vi "motionmenu.vi"(8 "Elements":string[](array[string]), 11 "NXT/EV3 2":T1) -> (0 "Goto":dbl, 1 "Continue?":bool, 3 "NXT/EV3":T1)   [LabVIEW 2013]
uses:
  <vilib>/NXT/Subs/LVHSConnector.ctl
  <vilib>/NXT/LegoClasses/BrickReference/BrickReference.lvclass
  <vilib>/NXT/Dual Mode Library/Waits/Wait_Num.vi
  <vilib>/NXT/Dual Mode Library/Display/clearDisplay.vi
  <vilib>/NXT/Dual Mode Library/Display/drawPicture.vi
  <vilib>/NXT/Dual Mode Library/Advanced/NXTFlag_Get.vi
  <vilib>/NXT/Dual Mode Library/Advanced/NXTFlag_Clear.vi
  <vilib>/NXT/Dual Mode Library/Advanced/NXTFlag_Get_Integer.vi
  <vilib>/NXT/Dual Mode Library/Sensors/EV3_Ultrasonic_CM.vi
  <vilib>/NXT/Dual Mode Library/Display/drawText_Center.vi
  <vilib>/NXT/Dual Mode Library/Advanced/NXTFlag_Assign.vi
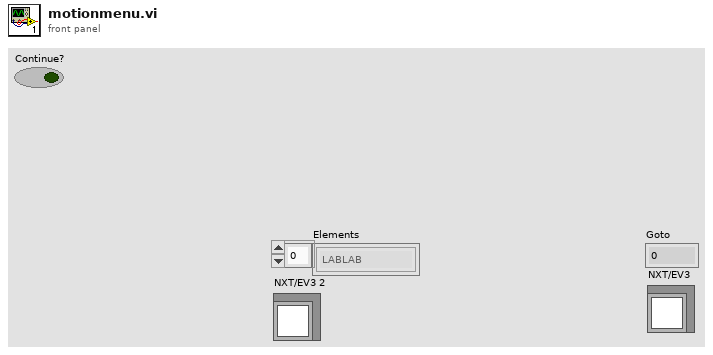
[diagram p1: front panel]
types:
  T1 = typedef "LVHSConnector.ctl" = refnum<class "BrickReference.lvclass">
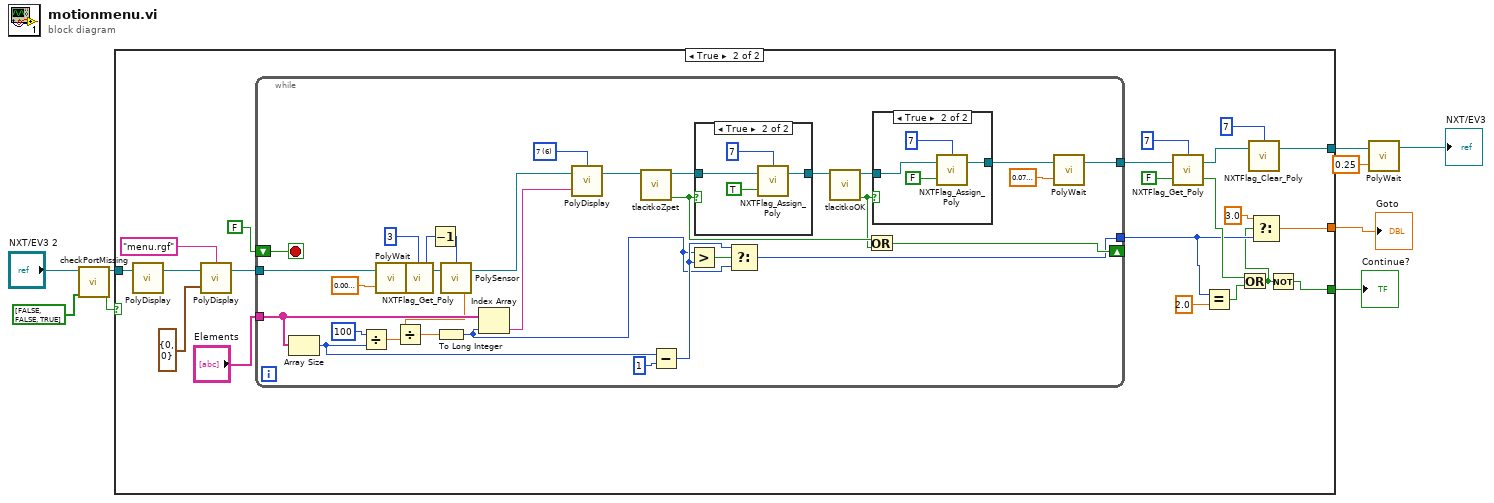
[diagram p0: block diagram]
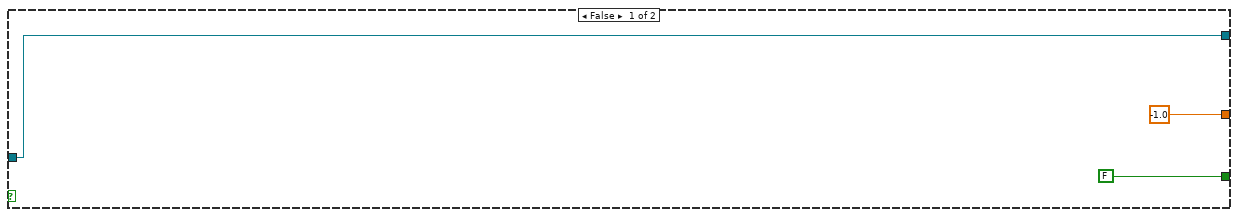
[diagram p2: hidden frame]
diagram:
  n1 = call "checkPortMissing.vi"("Required"=bool[] [FALSE, FALSE, TRUE], "NXT/EV3"="NXT/EV3 2") -> ("Success"=w4:bool, "NXT/EV3"=w6:T1)  [unwired: 8 in]
  n2 = case shown="True" w4 {
    tunnel: [-1.0 ("t") w18] -> w9
    tunnel: [w12 w21] -> w7
    tunnel: w6 -> [w12 w20]
    tunnel: [FALSE ("Boolean") w16] -> w3
    frame False {
    }
    frame True {
      n3 = call-poly <vilib>:"PolyDisplay.vi"("NXT/EV3"=w20) -> ("NXT/EV3"=w24:T1)  [unwired: 3 in]
      n4 = call-poly <vilib>:"PolyDisplay.vi"("Origin"=cluster{"X":i16, "Y":i16} {"X"=0, "Y"=0}, "NXT/EV3"=w24, "Filename (*.ric/*.rgf)"="menu.rgf") -> ("NXT/EV3"=w25:T1)  [unwired: 1 in]
      n5 = while {
        shift-right: [w60] -> _
        shift-left: FALSE -> [w61]
        tunnel: "Elements" -> [w64]
        tunnel: [w55] -> w31
        tunnel: [w46] -> w14
        tunnel: w25 -> [w57]
        stop <- w61 stop-if-true
        w62 = i16 6 items=["1", "2", "3", "4", "5", "6", "7", "8", "9", "10", "11", "12"] ("Line")
        n6 = Array Size(array=w64) -> (size(s)=w43:i32)
        n7 = Divide(x=100, y=w43) -> (x/y=w44:dbl)
        n8 = call-poly <vilib>:"PolyWait.vi"("Time (1 sec)"=sgl 0.01, "NXT/EV3"=w57) -> ("NXT/EV3"=w40:T1)  [unwired: 2 in]
        n9 = call-poly <vilib>:"NXTFlag_Get_Poly.vi"("NXT/EV3"=w40, "NXT/EV3 Flag Number"=3) -> ("Flag Value"=w36:i32, "NXT/EV3"=w37:T1)  [unwired: 1 in]
        n10 = Decrement(x=w36) -> (x-1=w34:i32)
        n11 = call-poly <vilib>:"PolySensor.vi"("NXT/EV3"=w37, "Port (Port 1)"=w34) -> ("Centimeters"=w38:sgl, "NXT/EV3"=w39:T1)  [unwired: 1 in]
        n12 = Divide(x=w38, y=w44) -> (x/y=w45:dbl)
        n13 = To Long Integer(number=w45) -> (32bit integer=w41:i32)
        n14 = Index Array(array=w64, index=w41) -> (element=w63:string)
        n15 = call-poly <vilib>:"PolyDisplay.vi"("Text"=w63, "NXT/EV3"=w39, "Line"=w62) -> ("NXT/EV3"=w50:T1)  [unwired: 1 in]
        n16 = call "tlacitkoZpet.vi"("NXT/EV3"=w50) -> ("Boolean"=w54:bool, "NXT/EV3 2"=w49:T1)  [unwired: 9 in]
        n17 = Subtract(x=w43, y=1) -> (x-y=w48:i32)
        n18 = Greater?(x=w41, y=w48) -> (0:w65:bool)
        n19 = case shown="True" w54 {
          tunnel: w49 -> [w71 w73]
          tunnel: [w71 w72] -> w52
          frame False {
          }
          frame True {
            n20 = call-poly <vilib>:"NXTFlag_Assign_Poly.vi"("Flag State"=TRUE, "NXT/EV3"=w73, "NXT/EV3 Flag Number"=i8 7) -> ("NXT/EV3"=w72:T1)  [unwired: 1 in]
          }
        }
        n21 = Select(t=w48, s=w65, f=w41) -> (s? t:f=w46:i32)
        n22 = call "tlacitkoOK.vi"("NXT/EV3"=w52) -> ("Boolean"=w53:bool, "NXT/EV3 2"=w51:T1)  [unwired: 9 in]
        n23 = Or(x=w54, y=w53) -> (x .or. y?=w60:bool)
        n24 = case shown="True" w53 {
          tunnel: w51 -> [w66 w68]
          tunnel: [w66 w67] -> w56
          frame False {
          }
          frame True {
            n25 = call-poly <vilib>:"NXTFlag_Assign_Poly.vi"("Flag State"=FALSE, "NXT/EV3"=w68, "NXT/EV3 Flag Number"=i8 7) -> ("NXT/EV3"=w67:T1)  [unwired: 1 in]
          }
        }
        n26 = call-poly <vilib>:"PolyWait.vi"("Time (1 sec)"=sgl 0.08, "NXT/EV3"=w56) -> ("NXT/EV3"=w55:T1)  [unwired: 2 in]
      }
      n27 = call-poly <vilib>:"NXTFlag_Get_Poly.vi"("Clear if Found"=FALSE, "NXT/EV3"=w31, "NXT/EV3 Flag Number"=7) -> ("status"=w15:bool, "NXT/EV3"=w27:T1)
      n28 = Equal?(x=w14, y=2.0) -> (x = y?=w19:bool)
      n29 = Or(x=w15, y=w19) -> (x .or. y?=w13:bool)
      n30 = call-poly <vilib>:"NXTFlag_Clear_Poly.vi"("NXT/EV3"=w27, "NXT/EV3 Flag Number"=7) -> ("NXT/EV3"=w21:T1)  [unwired: 2 in]
      n31 = Select(t=3.0, s=w13, f=w14) -> (s? t:f=w18:dbl)
      n32 = Not(x=w13) -> (.not. x?=w16:bool)
    }
  }
  "Goto" <- w9
  "Continue?" <- w3
  n33 = call-poly <vilib>:"PolyWait.vi"("Time (1 sec)"=sgl 0.25, "NXT/EV3"=w7) -> ("NXT/EV3"=→"NXT/EV3":T1)  [unwired: 2 in]
